vi "Initialize.vi"(8 "error in (no error)":errorcluster, 10 "shared resources":refnum<class "Shared Resources.lvclass">, 11 "Execution Unit Implementation in":refnum<class "Execution Unit.lvclass">) -> (0 "error out":errorcluster, 3 "Execution Unit Implementation out":refnum<class "Execution Unit.lvclass">)   [LabVIEW 2020, in "Communication Bus Template Engine.lvlib" / "Implementation.lvlib" / "Execution Unit.lvclass"]
uses:
  Execution Unit.lvclass
  Interfaces/Shared Resources/Shared Resources.lvclass
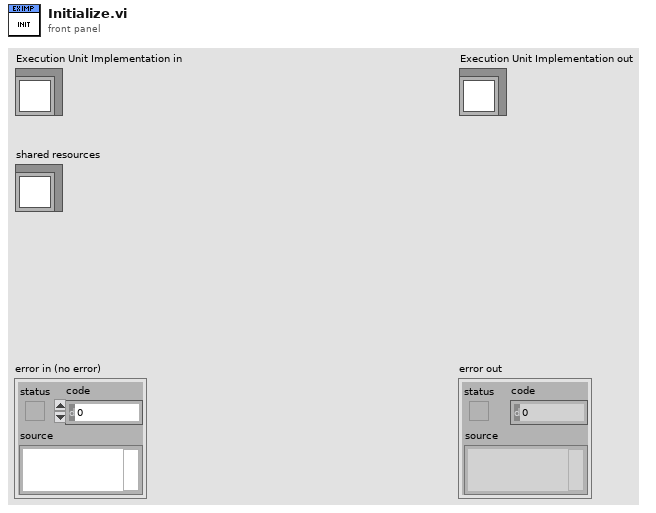
[diagram p1: front panel]
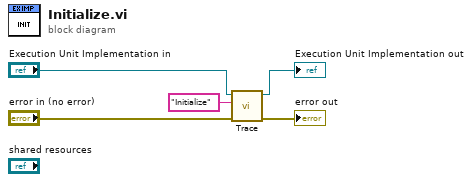
[diagram p0: block diagram]
diagram:
  n1 = call "Trace.vi"("Execution Unit Implementation in"="Execution Unit Implementation in", "message"="Initialize" ("input 2"), "error in (no error)"="error in (no error)") -> ("Execution Unit Implementation out"=→"Execution Unit Implementation out":refnum<class "Execution Unit.lvclass">, "error out"=→"error out":errorcluster)  [unwired: 6 in]
